vi "Octal Channel Write AOTF Config File.vi"() -> ()   [LabVIEW 2016]
uses:
  Octal Channel Type Defs/Octal Channel AOTF Config.ctl
panel:
  in  "AOTF Config":T1
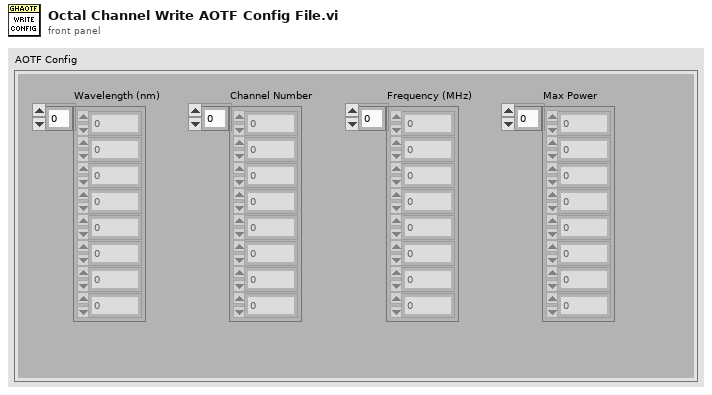
[diagram p1: front panel]
types:
  T1 = typedef "Octal Channel AOTF Config.ctl" = cluster{"Wavelength (nm)":u16[], "Channel Number":u8[], "Frequency (MHz)":dbl[], "Max Power":dbl[]}
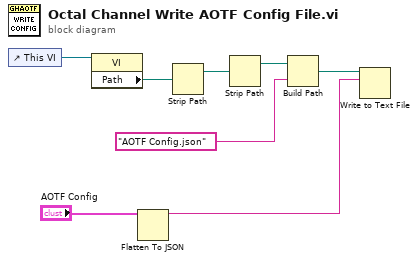
[diagram p0: block diagram]
diagram:
  n1 = control-ref of="This VI"() -> (w8:refnum<vi>)
  n2 = property class="VI"(reference=w8) -> ("Path"=w7:path)  [unwired: 1 in, 2 out]
  n3 = Flatten To JSON(anything="AOTF Config") -> (JSON string=w1:string)  [unwired: 2 in, 1 out]
  n4 = Strip Path(path=w7) -> (stripped path=w6:path)  [unwired: 1 out]
  n5 = Strip Path(path=w6) -> (stripped path=w5:path)  [unwired: 1 out]
  n6 = Build Path(base path=w5, name or relative path="AOTF Config.json") -> (appended path=w2:path)
  n7 = Write to Text File(file (use dialog)=w2, text=w1) -> ()  [unwired: 2 in, 3 out]
